vi "Check Temperatures.vi"(6 "lower limit (10C)":dbl=10.0, 7 "upper limit (100C)":dbl=100.0, 8 "error in (no error)":errorcluster, 10 "Container":T1, 11 "cRIO-CO2 in":refnum<class "cRIO-CO2.lvclass">) -> (0 "error out":errorcluster, 2 "In Range?":bool, 3 "cRIO-CO2 out":refnum<class "cRIO-CO2.lvclass">)   [LabVIEW 2015, in "cRIO-Carbondioxide.lvlib" / "cRIO-CO2.lvlib" / "cRIO-CO2.lvclass"]
uses:
  cRIO-CO2.lvclass
  Controls/Sample Transfer Container Enumerator.ctl
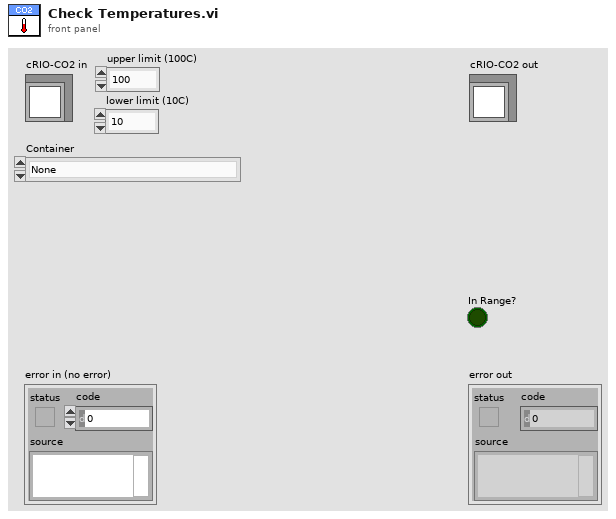
[diagram p1: front panel]
types:
  T1 = typedef "Sample Transfer Container Enumerator.ctl" = enum16{"None", "Sample 1", "Sample 2", "Sample 3", "Sample 4", "Sample 5", "Storage 01", "Storage 02", "Storage 03", "Storage 04", "Storage 05", "Storage 06", "Storage 07", "Storage 08", "Storage 09", "Storage 10", "Storage 11", "Storage 12", "Syringe", "Undefined"}
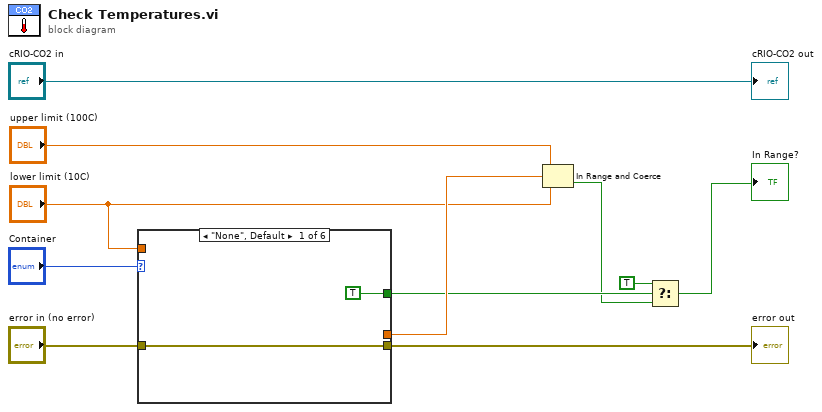
[diagram p0: block diagram]
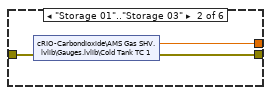
[diagram p2: hidden frame]
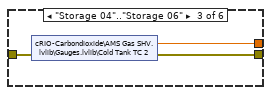
[diagram p3: hidden frame]
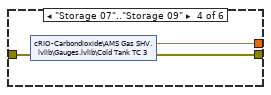
[diagram p4: hidden frame]
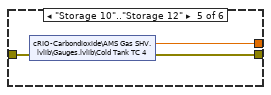
[diagram p5: hidden frame]
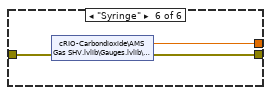
[diagram p6: hidden frame]
diagram:
  n1 = case shown="\"None\", Default" "Container" {
    tunnel: "error in (no error)" -> [w13 w16 w19 w22 w25 w28]
    tunnel: [w13 w15 w18 w21 w24 w27] -> w10
    tunnel: [_ w14 w17 w20 w23 w26] -> w6
    tunnel: "lower limit (10C)" -> [_ _ _ _ _ _]
    tunnel: [TRUE _ _ _ _ _] -> w4
    frame "None", Default {
    }
    frame "Storage 01".."Storage 03" {
      n2 = shared-variable "cRIO-Carbondioxide\\AMS Gas SHV.lvlib\\Gauges.lvlib\\Cold Tank TC 1"(error in=w16) -> (w14:dbl, error out=w15:errorcluster)
    }
    frame "Storage 04".."Storage 06" {
      n3 = shared-variable "cRIO-Carbondioxide\\AMS Gas SHV.lvlib\\Gauges.lvlib\\Cold Tank TC 2"(error in=w19) -> (w17:dbl, error out=w18:errorcluster)
    }
    frame "Storage 07".."Storage 09" {
      n4 = shared-variable "cRIO-Carbondioxide\\AMS Gas SHV.lvlib\\Gauges.lvlib\\Cold Tank TC 3"(error in=w22) -> (w20:dbl, error out=w21:errorcluster)
    }
    frame "Storage 10".."Storage 12" {
      n5 = shared-variable "cRIO-Carbondioxide\\AMS Gas SHV.lvlib\\Gauges.lvlib\\Cold Tank TC 4"(error in=w25) -> (w23:dbl, error out=w24:errorcluster)
    }
    frame "Syringe" {
      n6 = shared-variable "cRIO-Carbondioxide\\AMS Gas SHV.lvlib\\Gauges.lvlib\\Syringe TC"(error in=w28) -> (w26:dbl, error out=w27:errorcluster)
    }
  }
  "error out" <- w10
  n7 = In Range and Coerce(upper limit="upper limit (100C)", x=w6, lower limit="lower limit (10C)") -> (In Range?=w2:bool)  [unwired: 1 out]
  n8 = Select(t=TRUE, s=w4, f=w2) -> (s? t:f=→"In Range?":bool)
  "cRIO-CO2 out" <- "cRIO-CO2 in"
